vi "Counter - Read Encoder Velocity4 (Continuous Clock).vi"() -> ()   [LabVIEW 2015]
doc: "This example demonstrates how to use a counter input along with an external clock to continually sample the angular velocity measured from an encoder.\n\nFor instructions on how to connect your signals to the DAQ device, refer to your device documentation."
uses:
  <vilib>/Utility/error.llb/DialogType.ctl
  <vilib>/DAQmx/read.llb/DAQmx Read (Analog 1D Wfm NChan NSamp).vi
  <vilib>/DAQmx/read.llb/DAQmx Read (Counter 2D DBL NChan NSamp).vi
  <vilib>/DAQmx/create/channels.llb/DAQmx Create Channel (CI-Velocity-Linear).vi
  <vilib>/DAQmx/create/channels.llb/DAQmx Create Channel (AI-Voltage-Basic).vi
  <vilib>/DAQmx/configure/timing.llb/DAQmx Timing (Sample Clock).vi
  <vilib>/DAQmx/miscellaneous.llb/DAQmx Fill In Error Info.vi
  <resource>/objmgr/daqmx.rc
panel:
  in  "Channel 2":bool=TRUE
  in  "Channel 1":bool=TRUE
  out "appended path":path
  in  "Row 1 Header":string="Header Information Row 1"
  out "Boolean":bool
  out "Waveform Chart":dbl(graph)
  out "Numeric Indicator":dbl format="%.1g"
  in  "Counter 0":tag="Mantis1_1Mod4/ctr0"
  in  "B Input Terminal":tag="/Mantis1_1Mod4/PFI7"
  in  "A Input Terminal":tag="/Mantis1_1Mod4/PFI0"
  in  "Stop":bool
  in  "Samples per Loop":i32=1
  in  "Sample Rate":dbl=100.0
  in  "Sample Clock Source":tag="OnboardClock"
  # "MPH"
  # "Channel Settings"
  # "Saving data"
  # "Timing Settings"
  # "Trigger Rising Edge?"
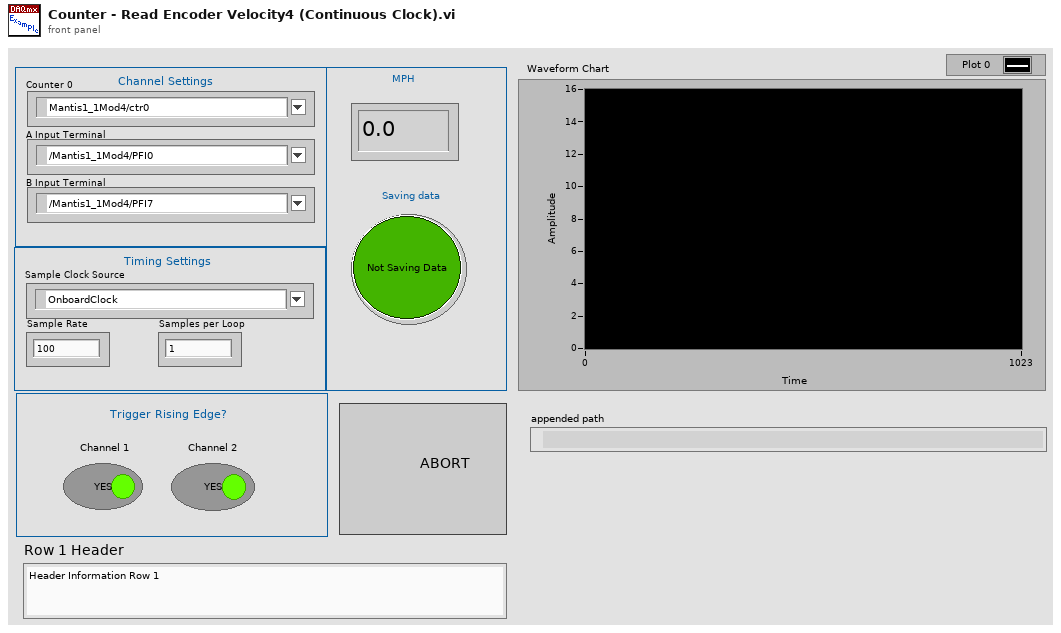
[diagram p1: front panel]
types:
  T1 = typedef "DialogType.ctl" = u16
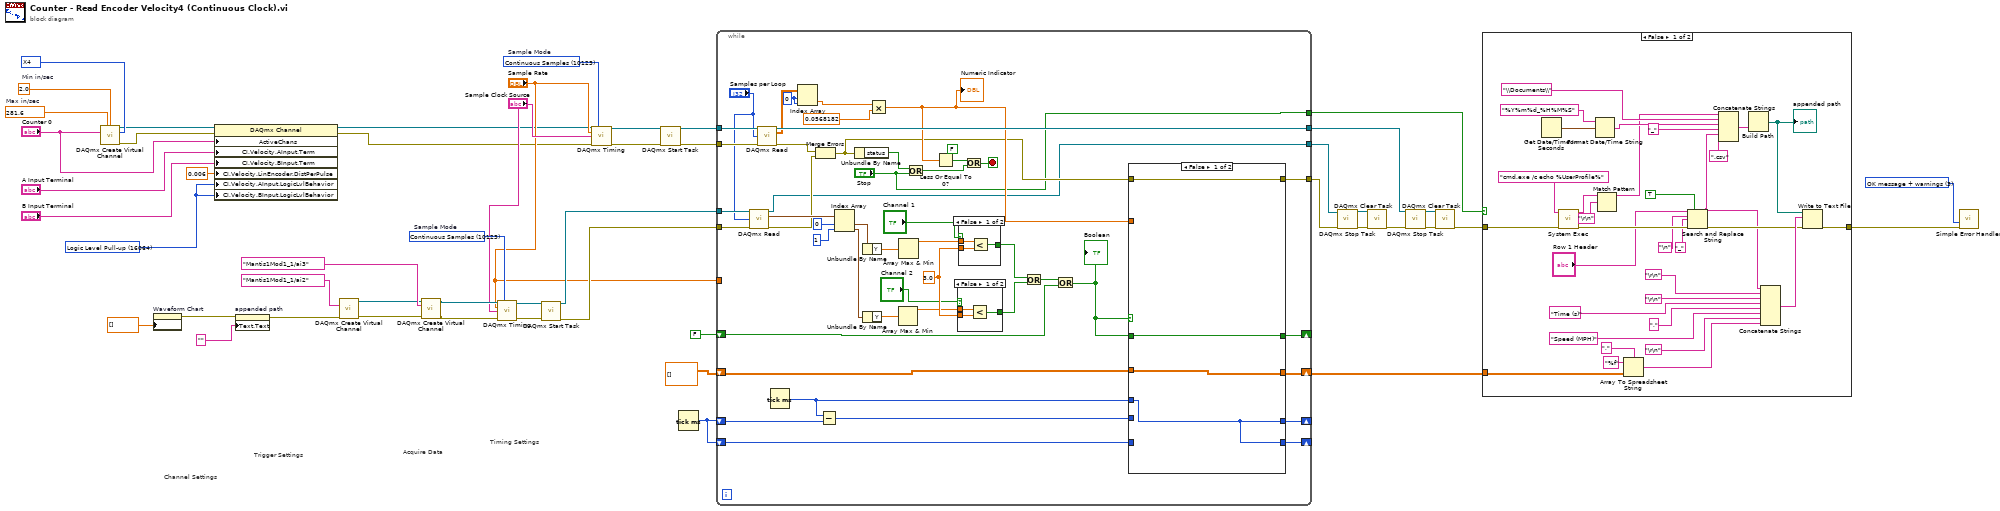
[diagram p0: block diagram]
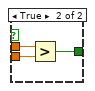
[diagram p3: hidden frame]
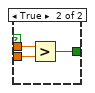
[diagram p4: hidden frame]
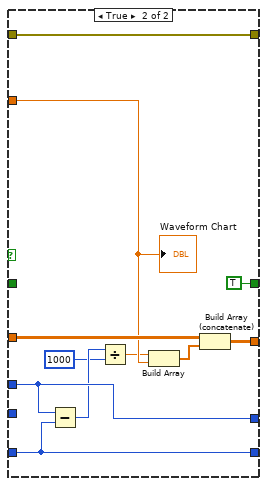
[diagram p5: hidden frame]
diagram:
  w2 = 16064 items=["Logic Level Pull-up"=16064, "None"=10230] ("CI.Velocity.AInput.LogicLvlBehavior")
  w31 = 10123 items=["Finite Samples"=10178, "Continuous Samples"=10123, "Hardware Timed Single Point"=12522]  # Sample Mode
  w44 = 281.6  # Max in/sec
  w43 = 2.0  # Min in/sec
  w38 = 10092 items=["X1"=10090, "X2"=10091, "X4"=10092, "Two Pulse Counting"=10313] ("decoding type")
  w45 = T1 3 items=["no dialog", "OK message", "continue or stop message", "OK message + warnings", "continue/stop + warnings"] ("type of dialog (OK msg:1)")
  w50 = 10123 items=["Finite Samples"=10178, "Continuous Samples"=10123, "Hardware Timed Single Point"=12522]  # Sample Mode
  # "Acquire Data"
  # "Trigger Settings"
  # "Timing Settings"
  # "Channel Settings"
  n1 = call-poly <vilib>:"DAQmx Create Virtual Channel.vi"("maximum value"=w44, "minimum value"=w43, "counter"="Counter 0", "decoding type"=w38) -> ("task out"=w6:refnum<k21>, "error out"=w5:errorcluster)  [unwired: 10 in]
  n2 = property on="Waveform Chart" class="WFChart (strict)"("History Data"=dbl[] []) -> (error out=w16:errorcluster)  [unwired: 2 in, 1 out]
  n3 = property class="DAQmx Channel"(reference=w6, error in=w5, "ActiveChans"="Counter 0", "CI.Velocity.AInput.Term"="A Input Terminal", "CI.Velocity.BInput.Term"="B Input Terminal", "CI.Velocity.LinEncoder.DistPerPulse"=0.006, "CI.Velocity.AInput.LogicLvlBehavior"=w2, "CI.Velocity.BInput.LogicLvlBehavior"=w2) -> (reference out=w3:refnum<k21>, error out=w4:errorcluster)
  n4 = property on="appended path" class="Path"(error in=w16, "Text.Text"="" ("Path Text.Text")) -> (error out=w15:errorcluster)  [unwired: 1 in, 1 out]
  n5 = call-poly <vilib>:"DAQmx Create Virtual Channel.vi"("physical channels"=tag "Mantis1Mod1_1/ai2", "error in"=w15) -> ("task out"=w35:refnum<k21>, "error out"=w34:errorcluster)  [unwired: 12 in]
  n6 = call-poly <vilib>:"DAQmx Create Virtual Channel.vi"("task in"=w35, "physical channels"=tag "Mantis1Mod1_1/ai3", "error in"=w34) -> ("task out"=w30:refnum<k21>, "error out"=w29:errorcluster)  [unwired: 11 in]
  n7 = call-poly <vilib>:"DAQmx Timing.vi"("task/channels in"=w30, "sample mode"=w31, "rate"="Sample Rate", "source"="Sample Clock Source", "error in"=w29) -> ("task out"=w27:refnum<k21>, "error out"=w26:errorcluster)  [unwired: 9 in]
  n8 = call <vilib>:"DAQmx Start Task.vi"("task/channels in"=w27, "error in"=w26) -> ("task out"=w24:refnum<k21>, "error out"=w23:errorcluster)  [unwired: 12 in]
  n9 = call-poly <vilib>:"DAQmx Timing.vi"("task/channels in"=w3, "sample mode"=w50, "rate"="Sample Rate", "source"="Sample Clock Source", "error in"=w4) -> ("task out"=w32:refnum<k21>, "error out"=w33:errorcluster)  [unwired: 9 in]
  n10 = call <vilib>:"DAQmx Start Task.vi"("task/channels in"=w32, "error in"=w33) -> ("task out"=w49:refnum<k21>, "error out"=w48:errorcluster)  [unwired: 12 in]
  n11 = Tick Count (ms)() -> (millisecond timer value=w17:u32)
  n12 = while {
    tunnel: w49 -> [w97]
    tunnel: w48 -> [w96]
    tunnel: [w95] -> w10
    tunnel: w24 -> [w79]
    tunnel: w23 -> [w78]
    tunnel: "Sample Rate" -> [_]
    shift-right: [w71] -> _
    shift-left: w17 -> [w70]
    shift-right: [w63] -> _
    shift-left: w17 -> [w64]
    shift-right: [w61] -> w20
    shift-left: dbl[][] [] -> [w62]
    tunnel: [w60] -> w8
    tunnel: [w57] -> w9
    tunnel: ["Stop"] -> w7
    shift-right: [w51] -> _
    shift-left: FALSE -> [w53]
    stop <- w76 stop-if-true
    (unwired) FALSE ("x")
    w88 = 3.0 ("y")
    w74 = 0 ("disabled index (col)")
    n13 = call-poly <vilib>:"DAQmx Read.vi"("task/channels in"=w79, "number of samples per channel"="Samples per Loop", "error in"=w78) -> ("task out"=w57:refnum<k21>, "data"=w91:waveform(dbl)[], "error out"=w68:errorcluster)  [unwired: 10 in]
    n14 = call-poly <vilib>:"DAQmx Read.vi"("task/channels in"=w97, "number of samples per channel"="Samples per Loop", "error in"=w96) -> ("task out"=w95:refnum<k21>, "data"=w93:dbl[][], "error out"=w67:errorcluster)  [unwired: 10 in]
    n15 = Tick Count (ms)() -> (millisecond timer value=w69:u32)
    n16 = Index Array(array=w93, index (row)=w74, index (col)=w74) -> (element=w73:dbl)
    n17 = Merge Errors(w67, w68) -> (w66:errorcluster)
    n18 = Subtract(x=w69, y=w70) -> (x-y=w65:u32)
    n19 = Index Array(array=w91, index #1=0 ("index"), index #2=1 ("index")) -> (element #1=w81:waveform(dbl), element #2=w84:waveform(dbl))
    n20 = Unbundle By Name(w66) -> ("status"=w94:bool)
    n21 = Unbundle By Name(w81) -> ("Y"=w82:dbl[])
    n22 = Unbundle By Name(w84) -> ("Y"=w85:dbl[])
    n23 = Multiply(x=w73, y=0.0568182) -> (x*y=w75:dbl)
    "Numeric Indicator" <- w75
    n24 = Array Max & Min(array=w85) -> (max value=w87:dbl)  [unwired: 3 out]
    n25 = Array Max & Min(array=w82) -> (max value=w86:dbl)  [unwired: 3 out]
    n26 = Or(x=w94, y="Stop") -> (x .or. y?=w77:bool)
    n27 = Less Or Equal To 0?(x=w75) -> (x <= 0?=w55:bool)
    n28 = case shown="False" "Channel 2" {
      tunnel: [w99 w103] -> w90
      tunnel: w88 -> [w100 w102]
      tunnel: w87 -> [w98 w101]
      frame False {
        n29 = Less?(x=w98, y=w100) -> (x < y?=w99:bool)
      }
      frame True {
        n30 = Greater?(x=w101, y=w102) -> (0:w103:bool)
      }
    }
    n31 = case shown="False" "Channel 1" {
      tunnel: [w106 w109] -> w89
      tunnel: w88 -> [w104 w108]
      tunnel: w86 -> [w105 w107]
      frame False {
        n32 = Less?(x=w105, y=w104) -> (x < y?=w106:bool)
      }
      frame True {
        n33 = Greater?(x=w107, y=w108) -> (0:w109:bool)
      }
    }
    n34 = Or(x=w55, y=w77) -> (x .or. y?=w76:bool)
    n35 = Or(x=w89, y=w90) -> (x .or. y?=w54:bool)
    n36 = Or(x=w54, y=w53) -> (x .or. y?=w52:bool)
    "Boolean" <- w52
    n37 = case shown="False" w52 {
      tunnel: w75 -> [_ w121]
      tunnel: w69 -> [w111 w119]
      tunnel: [w111 w119] -> w71
      tunnel: w66 -> [w112 w120]
      tunnel: w65 -> [_ _]
      tunnel: w64 -> [_ w118]
      tunnel: [w111 w118] -> w63
      tunnel: [w113 w123] -> w61
      tunnel: w62 -> [w113 w124]
      tunnel: [w112 w120] -> w60
      tunnel: [w110 TRUE] -> w51
      tunnel: w52 -> [w110 _]
      frame False {
      }
      frame True {
        n38 = Subtract(x=w119, y=w118) -> (x-y=w116:u32)
        n39 = Divide(x=w116, y=u32 1000) -> (x/y=w117:dbl)
        n40 = Build Array(w117, w121) -> (w122:dbl[])
        n41 = Build Array (concatenate)(w124, w122) -> (w123:dbl[][])
        "Waveform Chart" <- w121
      }
    }
  }
  n42 = call <vilib>:"DAQmx Stop Task.vi"("task/channels in"=w9, "error in"=w8) -> ("task out"=w13:refnum<k21>, "error out"=w12:errorcluster)  [unwired: 12 in]
  n43 = call <vilib>:"DAQmx Clear Task.vi"("task in"=w13, "error in"=w12) -> ("error out"=w11:errorcluster)  [unwired: 13 in]
  n44 = call <vilib>:"DAQmx Stop Task.vi"("task/channels in"=w10, "error in"=w11) -> ("task out"=w46:refnum<k21>, "error out"=w47:errorcluster)  [unwired: 12 in]
  n45 = call <vilib>:"DAQmx Clear Task.vi"("task in"=w46, "error in"=w47) -> ("error out"=w18:errorcluster)  [unwired: 13 in]
  n46 = case shown="False" w7 {
    tunnel: w20 -> [w151 _]
    tunnel: [w147 w157] -> w19
    tunnel: w18 -> [w137 w157]
    frame False {
      n47 = Get Date/Time In Seconds() -> (seconds since 1Jan1904=w145:timestamp)
      n48 = call <vilib>:"System Exec.vi"("error in (no error)"=w137, "command line"="cmd.exe /c echo %UserProfile%") -> ("error out"=w131:errorcluster, "standard output"=w136:string)  [unwired: 6 in, 2 out]
      n49 = Format Date/Time String(time format string (%c)="%Y%m%d_%H%M%S", seconds (now)=w145) -> (date/time string=w143:string)  [unwired: 1 out]
      n50 = Match Pattern(string=w136, regular expression="\r\n") -> (before substring=w135:string)  [unwired: 1 in, 3 out]
      n51 = Array To Spreadsheet String(delimiter (Tab)=",", array=w151, 3:"%f" ("format string")) -> (spreadsheet string=w148:string)
      n52 = Search and Replace String(replace all?=TRUE ("replace all? (F)"), input string="Row 1 Header", search string="\n", replace string="_" ("replace string (\"\")"), error in=w131) -> (result string=w128:string, error out=w130:errorcluster)  [unwired: 3 in, 2 out]
      n53 = Concatenate Strings(w135, "\\Documents\\" ("string"), w143, "_" ("string"), w128, ".csv" ("string")) -> (w142:string)
      n54 = Build Path(name or relative path=w142) -> (appended path=w141:path)  [unwired: 1 in]
      "appended path" <- w141
      n55 = Concatenate Strings(w128, "\r\n", "\r\n", "Time (s)", ",", "Speed (MPH)", "\r\n", w148) -> (w146:string)
      n56 = Write to Text File(file (use dialog)=w141, text=w146, error in=w130) -> (error out=w147:errorcluster)  [unwired: 1 in, 2 out]
    }
    frame True {
    }
  }
  n57 = call <vilib>:"Simple Error Handler.vi"("type of dialog (OK msg:1)"=w45, "error in (no error)"=w19) -> ()  [unwired: 3 in, 5 out]
